vi "Read Timer.vi"(8 "error in":errorcluster, 11 "Timer in":refnum<class "Timer.lvclass">) -> (0 "error out":errorcluster, 3 "Timer out":refnum<class "Timer.lvclass">)   [LabVIEW 2019, in "Timer.lvlib" / "Timer.lvclass"]
uses:
  Timer.lvclass
  C:/Program Files (x86)/National Instruments/LabVIEW 2019/vi.lib/ActorFramework/Actor/Actor.lvclass
  Timer.lvclass/Timer.ctl
  <vilib>/ActorFramework/Actor/Actor.lvclass/Actor.ctl
  Timer Messages/Time Info Msg/Time Info Msg.lvclass/Time Info Msg.ctl
  <vilib>/ActorFramework/Message Enqueuer/Message Enqueuer.lvclass/Message Enqueuer.ctl
  <vilib>/ActorFramework/Message Enqueuer/Enqueue.vi
  Timer Messages/Time Info Msg/Time Info Msg.lvclass
  C:/Program Files (x86)/National Instruments/LabVIEW 2019/vi.lib/ActorFramework/Message/Message.lvclass
  <vilib>/ActorFramework/Message Priority Queue/Priority Enqueue.vi
  <vilib>/ActorFramework/Actor/Actor.lvclass
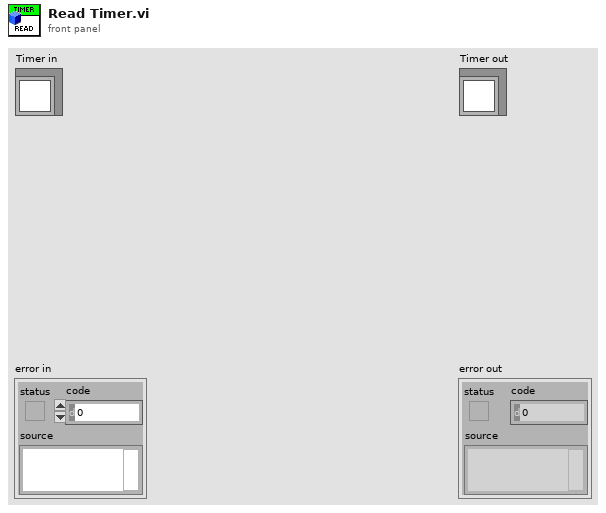
[diagram p1: front panel]
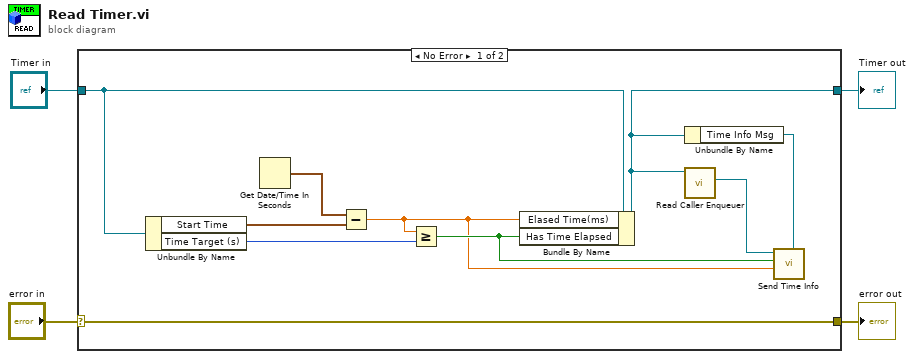
[diagram p0: block diagram]
diagram:
  n1 = case shown="No Error" "error in" {
    selector: "error in" -> [w14 w16]
    tunnel: [w14 w16] -> w3
    tunnel: [w10 w15] -> w1
    tunnel: "Timer in" -> [w13 w15]
    frame No Error {
      n2 = Unbundle By Name(w13) -> ("Start Time"=w12:timestamp, "Time Target (s)"=w11:i32)
      n3 = Get Date/Time In Seconds() -> (seconds since 1Jan1904=w9:timestamp)
      n4 = Subtract(x=w9, y=w12) -> (x-y=w5:dbl)
      n5 = Greater Or Equal?(x=w5, y=w11) -> (x >= y?=w6:bool)
      n6 = Bundle By Name(cluster=w13, "Elased Time(ms)"=w5, "Has Time Elapsed"=w6) -> (w10:refnum<class "Timer.lvclass">)
      n7 = Unbundle By Name(w10) -> ("Time Info Msg"=w8:refnum<class "Time Info Msg.lvclass">)
      n8 = call <vilib>:"Read Caller Enqueuer.vi"("Actor"=w10) -> ("Caller Enqueuer"=w7:refnum<class "Message Enqueuer.lvclass">)  [unwired: 10 in]
      n9 = call "Send Time Info.vi"("Message Type"=w8, "Elapsed Time"=w5, "Elapsed?"=w6, "Message Enqueuer"=w7) -> ()  [unwired: 6 in, 2 out]
    }
    frame Error {
    }
  }
  "error out" <- w3
  "Timer out" <- w1
